vi "Advanced Fit.vi"(4 "Offset":dbl format="%#_13g", 6 "Sinusoidal Fit Controls.Stat.":T1=enum."Ind. Traces", 8 "error in (no error)":errorcluster, 9 "Response":dbl[][](array[numeric]), 10 "Stimulus":dbl[][](array[numeric]), 11 "Halfwave Sinusoidal Fit in":refnum<class "Halfwave Sinusoidal Fit.lvclass">) -> (0 "error out":errorcluster, 2 "Gain and Phase out":T2 {"Phase SD" format="%.1f"; "Phase" format="%.1f"; "Gain SD" format="%.2f"; "Gain" format="%.2f"}, 3 "Halfwave Sinusoidal Fit out":refnum<class "Halfwave Sinusoidal Fit.lvclass">)   [LabVIEW 2016, in "Halfwave Sinusoidal Fit.lvclass"]
uses:
  Halfwave Sinusoidal Fit.lvclass
  gain and phase/Typedef - Gain and Phase.ctl
  gain and phase/Typedef_StatisticType.ctl
  Halfwave Sinusoidal Fit.lvclass/Halfwave Sinusoidal Fit.ctl
  Sinusoidal Fit.lvclass
  comm/nan operations/nan operations.lvlib
panel:
  # "Gain:"
  # "+/-"
  # "Phase:"
  # "+/-"
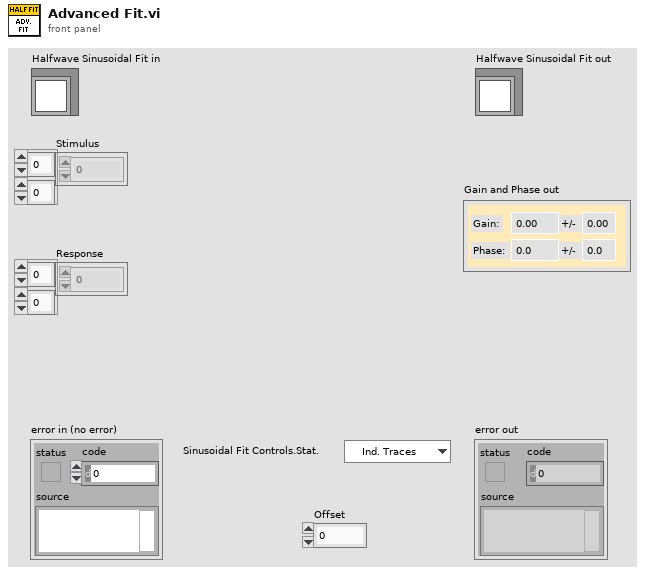
[diagram p1: front panel]
types:
  T1 = typedef "Typedef_StatisticType.ctl" = enum16{"Mean Trace", "Ind. Traces"}
  T2 = typedef "Typedef - Gain and Phase.ctl" = cluster{"Gain":dbl, "Gain SD":dbl, "Phase":dbl, "Phase SD":dbl}
  T3 = typedef "Typedef - Sinusoidal Fit Coefficients.ctl" = cluster{"Offset":dbl, "Gain":dbl, "Phase":dbl, "Freq":dbl}
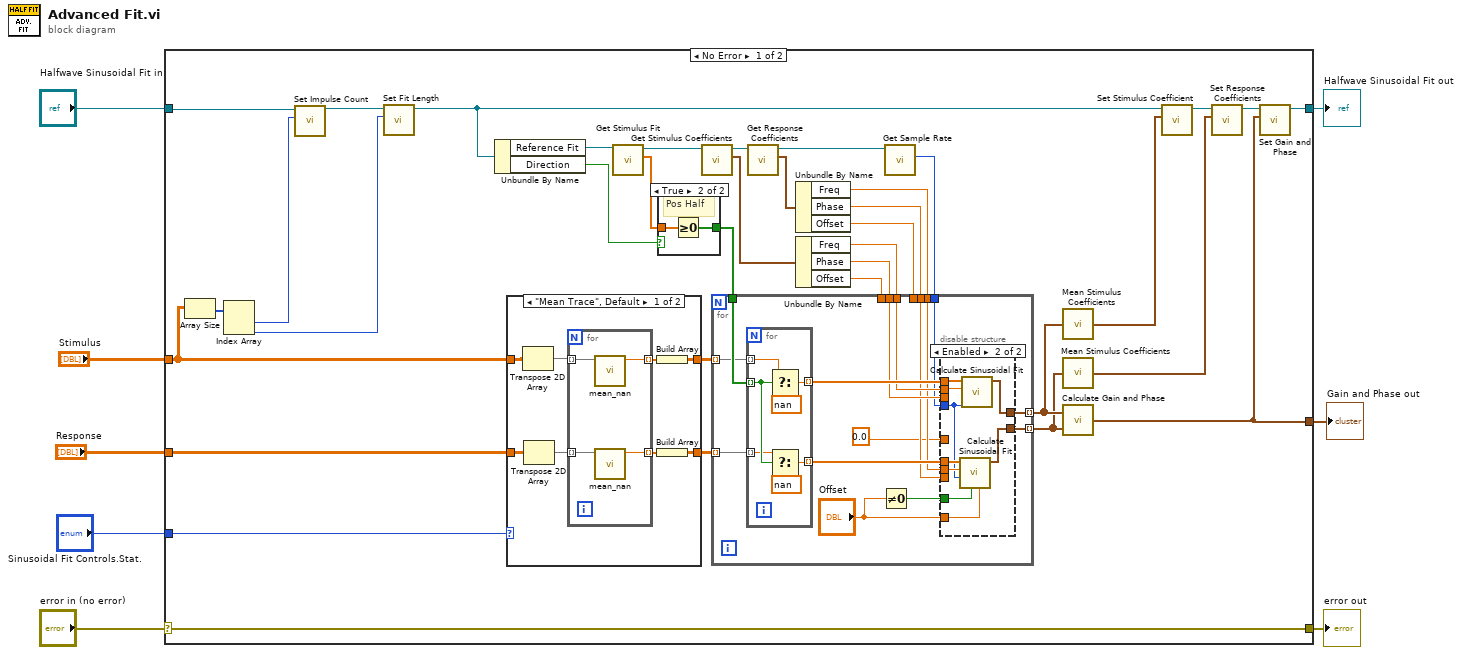
[diagram p0: block diagram]
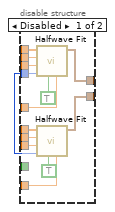
[diagram p3: hidden frame]
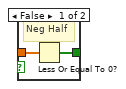
[diagram p4: hidden frame]
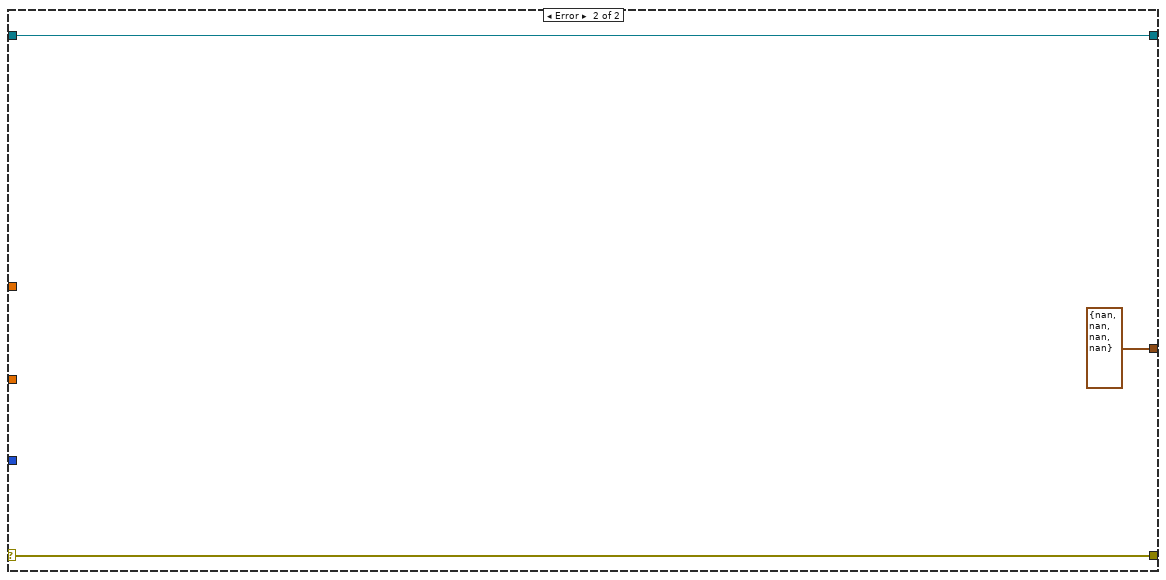
[diagram p5: hidden frame]
diagram:
  n1 = case shown="No Error" "error in (no error)" {
    selector: "error in (no error)" -> [w44 w108]
    tunnel: [w44 w108] -> w7
    tunnel: [w25 w107] -> w5
    tunnel: "Halfwave Sinusoidal Fit in" -> [w12 w107]
    tunnel: "Stimulus" -> [w16 _]
    tunnel: "Response" -> [w28 _]
    tunnel: "Sinusoidal Fit Controls.Stat." -> [w23 _]
    tunnel: [w18 T2 {"Gain"=nan, "Gain SD"=nan, "Phase"=nan, "Phase SD"=nan} ("Gain and Phase out")] -> w1
    frame No Error {
      n2 = Array Size(array=w16) -> (size(s)=w17:i32[])
      n3 = Index Array(array=w17) -> (element #1=w15:i32, element #2=w11:i32)  [unwired: 2 in]
      n4 = call-dynamic "Set Impulse Count.vi"("Nr of Fit Impulses"=w15, "Abstract Fit in"=w12) -> ("Abstract Fit out"=w13:refnum<class "Halfwave Sinusoidal Fit.lvclass">)  [unwired: 8 in, 1 out]
      n5 = call-dynamic "Set Fit Length.vi"("Length"=w11, "Abstract Fit in"=w13) -> ("Abstract Fit out"=w14:refnum<class "Halfwave Sinusoidal Fit.lvclass">)  [unwired: 8 in, 1 out]
      n6 = Unbundle By Name(w14) -> ("Reference Fit"=w31:refnum<class "Sinusoidal Fit.lvclass">, "Direction"=w24:bool)
      n7 = case shown="\"Mean Trace\", Default" w23 {
        tunnel: [w48 w58] -> w41
        tunnel: [w46 w57] -> w40
        tunnel: w16 -> [w51 w58]
        tunnel: w28 -> [w49 w57]
        frame "Mean Trace", Default {
          n8 = Transpose 2D Array(2D array=w51) -> (transposed array=w52:dbl[][])
          n9 = Transpose 2D Array(2D array=w49) -> (transposed array=w50:dbl[][])
          n10 = for {
            tunnel: [w56] -> w47 mode=indexing
            tunnel: [w55] -> w45 mode=indexing
            tunnel: w52 -> [w54] mode=indexing
            tunnel: w50 -> [w53] mode=indexing
            n11 = call "mean_nan.vi"("Array"=w54) -> ("Mean"=w56:dbl)  [unwired: 10 in]
            n12 = call "mean_nan.vi"("Array"=w53) -> ("Mean"=w55:dbl)  [unwired: 10 in]
          }
          n13 = Build Array(w47) -> (w48:dbl[][])
          n14 = Build Array(w45) -> (w46:dbl[][])
        }
        frame "Ind. Traces" {
        }
      }
      n15 = call-dynamic "Get Stimulus Fit.vi"("Sinusoidal Fit in"=w31) -> ("Fit out"=w43:dbl[], "Sinusoidal Fit out"=w39:refnum<class "Sinusoidal Fit.lvclass">)  [unwired: 8 in, 1 out]
      n16 = case shown="True" w24 {
        tunnel: w43 -> [w102 w105]
        tunnel: [w103 w104] -> w42
        frame False {
          # "Neg Half"
          n17 = Less Or Equal To 0?(x=w102) -> (x <= 0?=w103:bool[])
        }
        frame True {
          # "Pos Half"
          n18 = Greater Or Equal To 0?(x=w105) -> (x >= 0?=w104:bool[])
        }
      }
      n19 = call-dynamic "Get Stimulus Coefficients.vi"("Sinusoidal Fit in"=w39) -> ("Coefficients"=w38:T3, "Sinusoidal Fit out"=w35:refnum<class "Sinusoidal Fit.lvclass">)  [unwired: 8 in, 1 out]
      n20 = call-dynamic "Get Response Coefficients.vi"("Sinusoidal Fit in"=w35) -> ("Coefficients"=w34:T3, "Sinusoidal Fit out"=w30:refnum<class "Sinusoidal Fit.lvclass">)  [unwired: 8 in, 1 out]
      n21 = Unbundle By Name(w34) -> ("Freq"=w33:dbl, "Phase"=w32:dbl, "Offset"=w10:dbl)
      n22 = Unbundle By Name(w38) -> ("Freq"=w37:dbl, "Phase"=w36:dbl, "Offset"=w9:dbl)
      n23 = call-dynamic "Get Sample Rate.vi"("Abstract Fit in"=w30) -> ("Sample Rate"=w29:i32)  [unwired: 8 in, 2 out]
      n24 = for {
        tunnel: w42 -> [w73]
        tunnel: w41 -> [w72] mode=indexing
        tunnel: w40 -> [w71] mode=indexing
        tunnel: w37 -> [w68]
        tunnel: w36 -> [w67]
        tunnel: w33 -> [w66]
        tunnel: w32 -> [w65]
        tunnel: w29 -> [w64]
        tunnel: [w63] -> w22 mode=indexing
        tunnel: [w62] -> w20 mode=indexing
        tunnel: w10 -> [_]
        tunnel: w9 -> [_]
        n25 = for {
          tunnel: w73 -> [w98] mode=indexing
          tunnel: w72 -> [w101] mode=indexing
          tunnel: w71 -> [w97] mode=indexing
          tunnel: [w96] -> w69 mode=indexing
          tunnel: [w95] -> w70 mode=indexing
          n26 = Select(t=w101, s=w98, f=nan) -> (s? t:f=w96:dbl)
          n27 = Select(t=w97, s=w98, f=nan) -> (s? t:f=w95:dbl)
        }
        n28 = Not Equal To 0?(x="Offset") -> (x != 0?=w60:bool)
        n29 = disable-structure shown="Enabled" {
          disable-tunnel: w70 -> [w85 w91]
          disable-tunnel: w69 -> [w84 w94]
          disable-tunnel: w68 -> [w83 w93]
          disable-tunnel: w67 -> [w82 _]
          disable-tunnel: w66 -> [w81 w90]
          disable-tunnel: w65 -> [w80 _]
          disable-tunnel: w64 -> [w79 w89]
          disable-tunnel: [w78 w92] -> w63
          disable-tunnel: [w77 w88] -> w62
          disable-tunnel: 0.0 -> [w74 _]
          disable-tunnel: "Offset" -> [_ w87]
          disable-tunnel: w60 -> [_ w86]
          frame Disabled {
            n30 = call "Halfwave Fit.vi"("Offset"=w74, "Ignore Offset"=TRUE, "Sample Rate"=w79, "Phase (deg)"=w82, "Stimulus\nFrequency"=w83, "Data in"=w84) -> ("Coefficients"=w78:T3)  [unwired: 4 in, 1 out]
            n31 = call "Halfwave Fit.vi"("Offset"=w74, "Ignore Offset"=TRUE, "Sample Rate"=w79, "Phase (deg)"=w80, "Stimulus\nFrequency"=w81, "Data in"=w85) -> ("Coefficients"=w77:T3)  [unwired: 4 in, 1 out]
          }
          frame Enabled {
            n32 = call "Calculate Sinusoidal Fit.vi"("Offset"=w87, "Ignore Offset"=w86, "Sample Rate"=w89, "Stimulus\nFrequency"=w90, "Data in"=w91) -> ("Coefficients"=w88:T3)  [unwired: 5 in, 1 out]
            n33 = call "Calculate Sinusoidal Fit.vi"("Sample Rate"=w89, "Stimulus\nFrequency"=w93, "Data in"=w94) -> ("Coefficients"=w92:T3)  [unwired: 7 in, 1 out]
          }
        }
      }
      n34 = call "Mean Stimulus Coefficients.vi"("Coefficients in"=w22) -> ("Mean Coefficients out"=w21:T3)
      n35 = call "Mean Stimulus Coefficients.vi"("Coefficients in"=w20) -> ("Mean Coefficients out"=w19:T3)
      n36 = call "Calculate Gain and Phase.vi"("Response"=w20, "Stimulus"=w22) -> ("Gain and Phase out"=w18:T2)
      n37 = call-dynamic "Set Stimulus Coefficient.vi"("Coefficients"=w21, "Sinusoidal Fit in"=w14) -> ("Sinusoidal Fit out"=w27:refnum<class "Halfwave Sinusoidal Fit.lvclass">)  [unwired: 8 in, 1 out]
      n38 = call-dynamic "Set Response Coefficients.vi"("Coefficients"=w19, "Sinusoidal Fit in"=w27) -> ("Sinusoidal Fit out"=w26:refnum<class "Halfwave Sinusoidal Fit.lvclass">)  [unwired: 8 in, 1 out]
      n39 = call-dynamic "Set Gain and Phase.vi"("Gain and Phase"=w18, "Sinusoidal Fit in"=w26) -> ("Sinusoidal Fit out"=w25:refnum<class "Halfwave Sinusoidal Fit.lvclass">)  [unwired: 8 in, 1 out]
    }
    frame Error {
    }
  }
  "error out" <- w7
  "Halfwave Sinusoidal Fit out" <- w5
  "Gain and Phase out" <- w1
